vi "Verificacion_calibracion_host.vi"() -> ()   [LabVIEW 2015]
uses:
  <vilib>/Analysis/5stat.llb/RMS (DBL).vi
  <vilib>/Analysis/baseanly.llb/Mean (DBL).vi
  <vilib>/measure/madcrms.llb/Basic Averaged DC-RMS for 1 Chan.vi
  <vilib>/measure/maspectr.llb/FFT Spectrum (Mag-Phase) for 1 Chan.vi
  <vilib>/measure/NI_MAPro.lvlib
  <vilib>/Analysis/NI_AALPro.lvlib
  <vilib>/Analysis/NI_AALBase.lvlib
panel:
  in  "file (use dialog)":path
  in  "Canales a calibrar (4 o 8)":u32=8
  in  "Frecuencia de muestreo":dbl=25600.0
  in  "Nº del canal":i32
  in  "Aceleración del patrón (g RMS)":dbl=1.0
  in  "Frecuencia del patrón (Hz)":dbl=159.744
  out "RMS conseguido":dbl format="%0.2f"
  out "Waveform Graph 2":cluster{"f0":dbl, "df":dbl, "magnitude":dbl[]}(graph)
  out "Waveform Graph":waveform(dbl)[](graph)
  out "Frecuencia de excitación\nVibrómetro  (Hz)":dbl
  in  "Parámetro de sensibilidad\n           (mV/g)":sgl=10.0
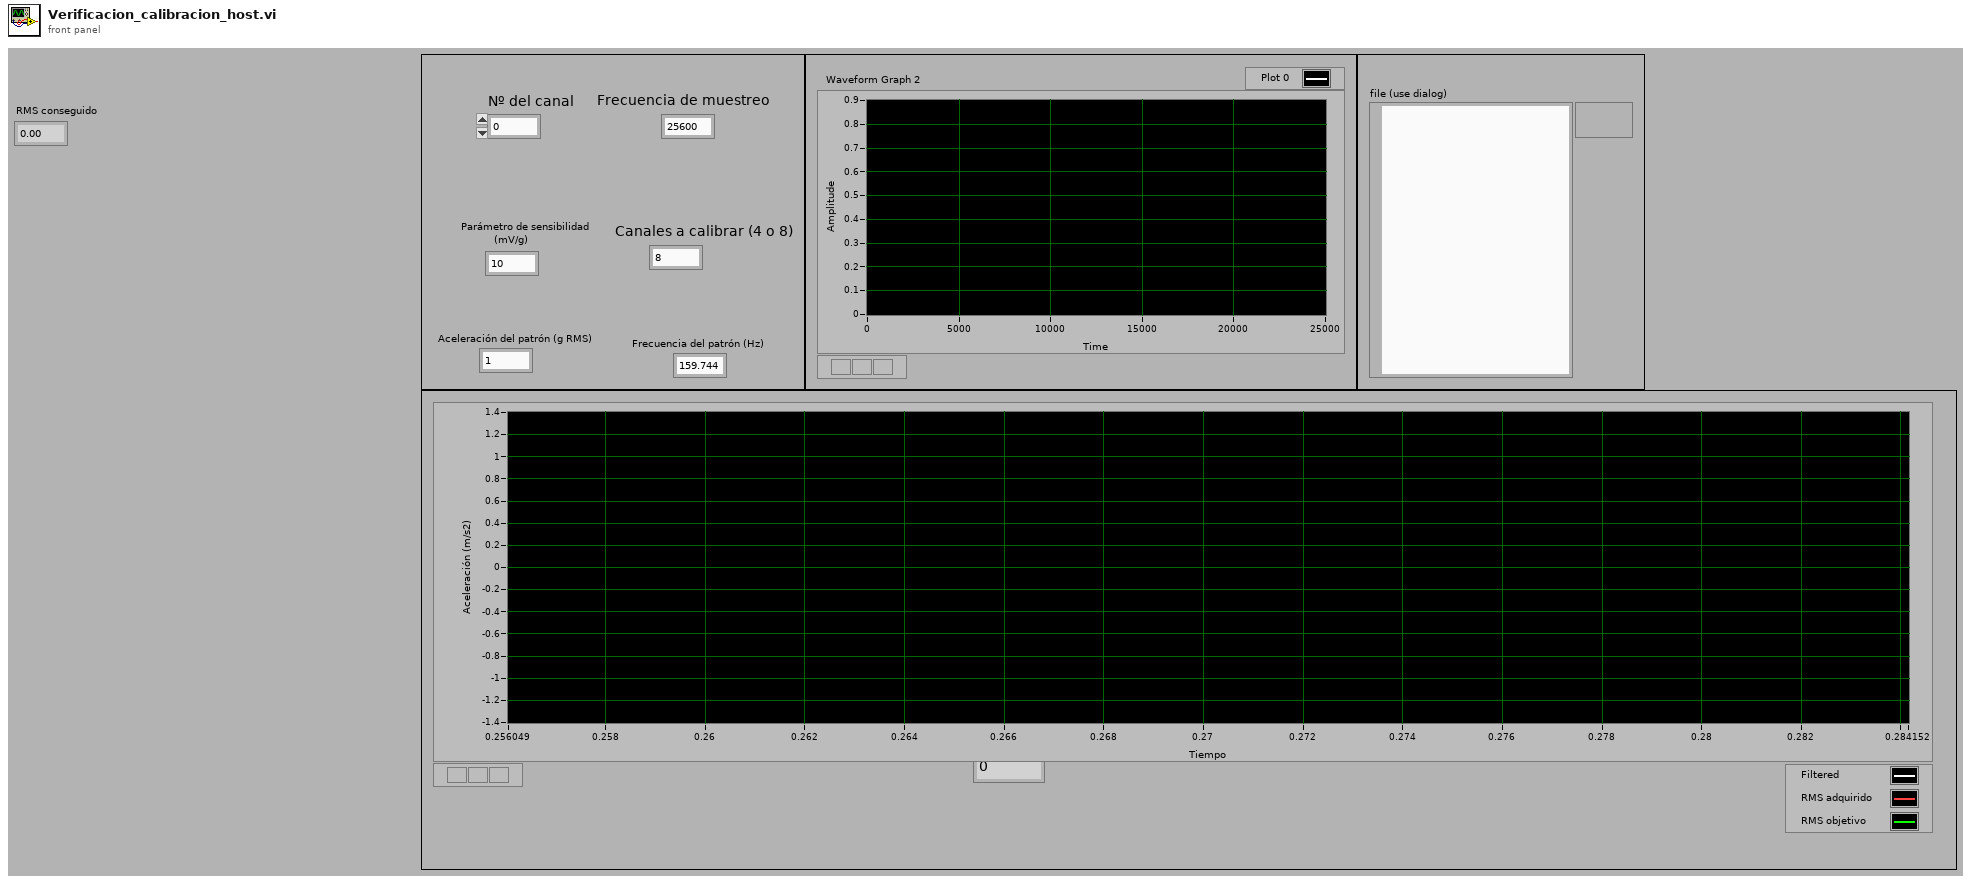
[diagram p1: front panel]
types:
  T1 = enum16{"big-endian, network order", "native, host order", "little-endian"}
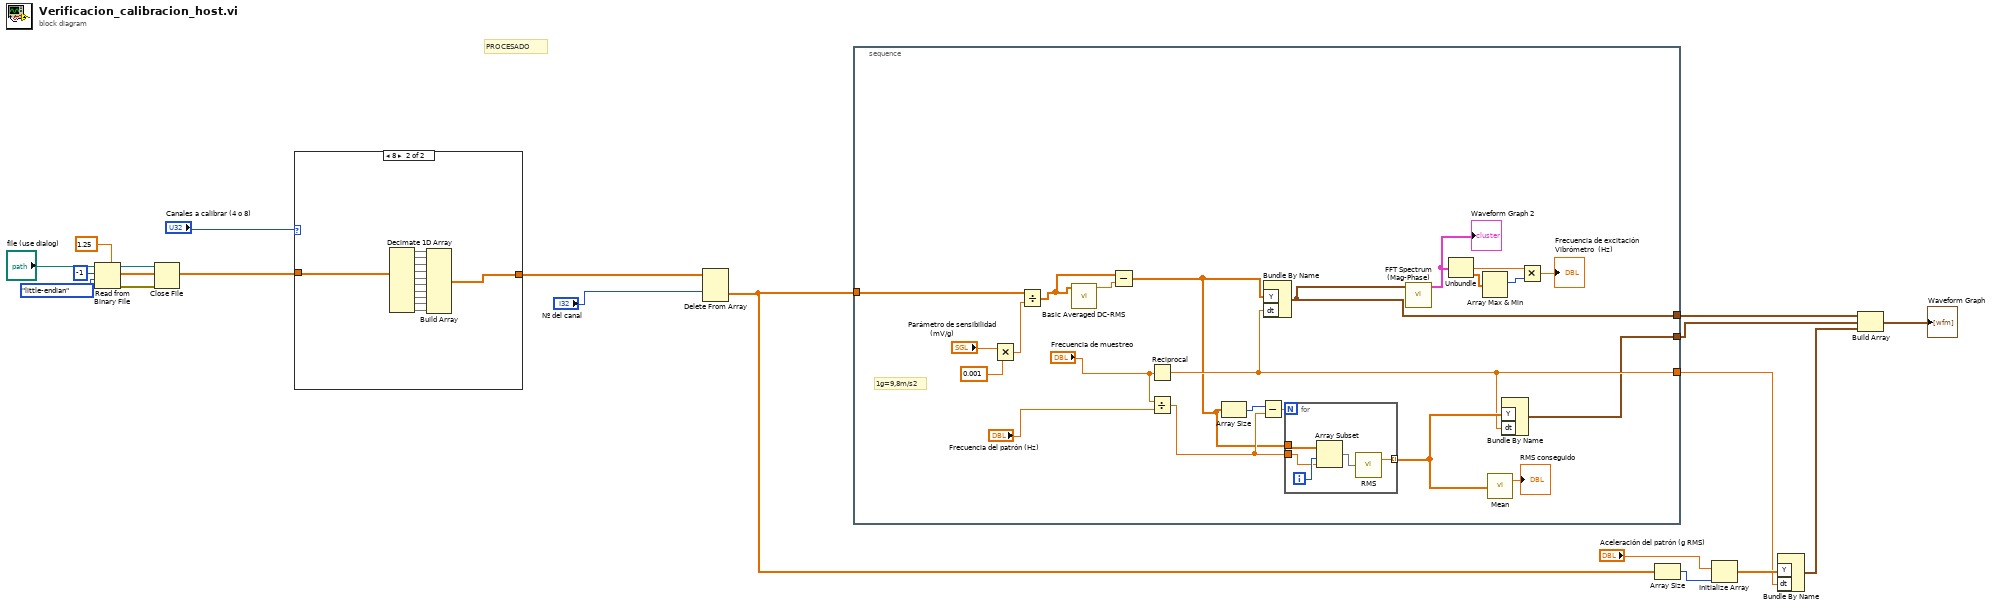
[diagram p0: block diagram]
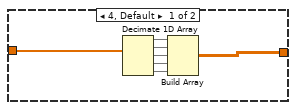
[diagram p2: hidden frame]
diagram:
  # "PROCESADO"
  n1 = Read from Binary File(5:sgl 1.25, 9:T1."little-endian" ("byte order (0:big-endian, network order)"), 10:-1 ("count (1)"), 11:"file (use dialog)") -> (0:w19:errorcluster, 2:w14:sgl[], 3:w16:refnum<file>)  [unwired: 1 in, 2 out]
  n2 = Close File(refnum=w16, error in=w19) -> ()  [unwired: 2 out]
  n3 = case shown="8" "Canales a calibrar (4 o 8)" {
    tunnel: w14 -> [w23 w35]
    tunnel: [w22 w34] -> w13
    frame 4, Default {
      n4 = Decimate 1D Array(w23) -> (w25:sgl[], w26:sgl[], w24:sgl[], w21:sgl[], w20:sgl[])
      n5 = Build Array(w25, w26, w24, w21, w20) -> (w22:sgl[][])
    }
    frame 8 {
      n6 = Decimate 1D Array(w35) -> (w37:sgl[], w38:sgl[], w36:sgl[], w30:sgl[], w29:sgl[], w31:sgl[], w32:sgl[], w33:sgl[], w28:sgl[], w27:sgl[])
      n7 = Build Array(w37, w38, w36, w30, w29, w31, w32, w33, w28, w27) -> (w34:sgl[][])
    }
  }
  n8 = Delete From Array(array=w13, index (row)="Nº del canal") -> (deleted portion=w7:sgl[])  [unwired: 2 in, 1 out]
  n9 = stacked-sequence {
    tunnel: [w39] -> w12
    tunnel: [w43] -> w9
    tunnel: w7 -> [w51]
    tunnel: [w41] -> w4
    frame #0 {
      # "1g=9,8m/s2"
      n10 = Multiply(x="Parámetro de sensibilidad\n           (mV/g)", y=0.001) -> (x*y=w55:dbl)
      n11 = Divide(x=w51, y=w55) -> (x/y=w50:dbl[])
      n12 = call-poly <vilib>:"Basic Averaged DC-RMS.vi"("signal in"=w50) -> ("DC value"=w53:dbl)  [unwired: 7 in, 3 out]
      n13 = Subtract(x=w50, y=w53) -> (x-y=w42:dbl[])
      n14 = Reciprocal(x="Frecuencia de muestreo") -> (1/x=w43:dbl)
      n15 = Divide(x="Frecuencia de muestreo", y="Frecuencia del patrón (Hz)") -> (x/y=w47:dbl)
      n16 = Array Size(array=w42) -> (size(s)=w48:i32)
      n17 = Subtract(x=w48, y=w47) -> (x-y=w49:dbl)
      n18 = Bundle By Name("Y"=w42, "dt"=w43) -> (w39:waveform(dbl))  [unwired: 1 in]
      n19 = for {
        N: w49 -> [_]
        tunnel: w47 -> [w62]
        tunnel: [w65] -> w46 mode=indexing
        tunnel: w42 -> [w64]
        i -> [w63]
        n20 = Array Subset(array=w64, index=w63, length=w62) -> (w61:dbl[])
        n21 = call-poly <vilib>:"RMS.vi"("X"=w61) -> ("rms value"=w65:dbl)  [unwired: 1 out]
      }
      n22 = call-poly <vilib>:"FFT Spectrum (Mag-Phase).vi"("time signal"=w39) -> ("magnitude"=w56:cluster{"f0":dbl, "df":dbl, "magnitude":dbl[]})  [unwired: 6 in, 4 out]
      "Waveform Graph 2" <- w56
      n23 = Unbundle(w56) -> ("df"=w58:dbl, "magnitude"=w59:dbl[])  [unwired: 1 out]
      n24 = Array Max & Min(array=w59) -> (max index (indices)=w60:i32)  [unwired: 3 out]
      n25 = call-poly <vilib>:"Mean.vi"("X"=w46) -> ("mean"=→"RMS conseguido":dbl)  [unwired: 1 out]
      n26 = Bundle By Name("Y"=w46, "dt"=w43) -> (w41:waveform(dbl))  [unwired: 1 in]
      n27 = Multiply(x=w58, y=w60) -> (x*y=→"Frecuencia de excitación\nVibrómetro  (Hz)":dbl)
    }
  }
  n28 = Array Size(array=w7) -> (size(s)=w11:i32)
  n29 = Initialize Array("Aceleración del patrón (g RMS)", w11) -> (w10:dbl[])
  n30 = Bundle By Name("Y"=w10, "dt"=w9) -> (w6:waveform(dbl))  [unwired: 1 in]
  n31 = Build Array(w12, w4, w6) -> (→"Waveform Graph":waveform(dbl)[])
